vi "Relace Hyfen - with _ underscore.vi"(11 "String include Hyfen'-'":string) -> (3 "string '-' Replace by '_' Underscore":string)   [LabVIEW 2021]
doc: "string '-' Replace by '_' Underscore"
uses:
  <userlib>/_OpenG.lib/array/array.llb/Search 1D Array (U8)__ogtk.vi
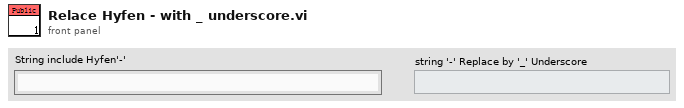
[diagram p1: front panel]
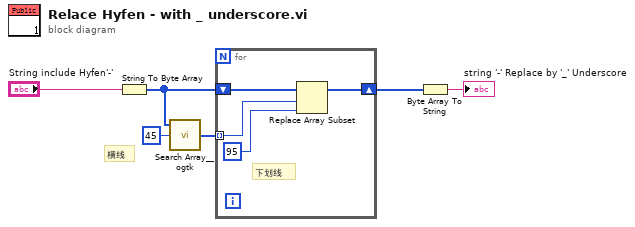
[diagram p0: block diagram]
diagram:
  # "横线"
  n1 = String To Byte Array(string="String include Hyfen'-'") -> (unsigned byte array=w5:u8[])
  n2 = call-poly <userlib>:"Search Array__ogtk.vi"("Array"=w5, "Element Data"=u8 45) -> ("Indices of Elements"=w4:i32[])  [unwired: 7 in]
  n3 = for {
    tunnel: w4 -> [w9] mode=indexing
    shift-right: [w7] -> w6
    shift-left: w5 -> [w10]
    # "下划线"
    n4 = Replace Array Subset(array=w10, new element=u8 95 ("new element/subarray"), index=w9) -> (w7:u8[])
  }
  n5 = Byte Array To String(unsigned byte array=w6) -> (string=→"string '-' Replace by '_' Underscore":string)
